vi "Read Unified Msg Set.vi"(11 "Base Setup in":refnum<class "Base Setup.lvclass">) -> (2 "Unified Msg Set":T1)   [LabVIEW 2025, in "jettl.lvlib" / "Setup.lvlib" / "Base Setup.lvclass"]
uses:
  Base Setup.lvclass
  Msg Set.ctl
  Msg/Msg.lvclass
  Base Setup.lvclass/Base Setup.ctl
  jettl.lvlib
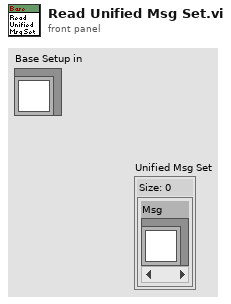
[diagram p1: front panel]
types:
  T1 = typedef "jettl.lvlib/Msg Set.ctl" = set{refnum<class "Msg.lvclass">}
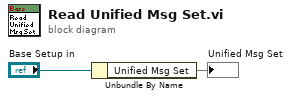
[diagram p0: block diagram]
diagram:
  n1 = Unbundle By Name("Base Setup in") -> ("Unified Msg Set"=→"Unified Msg Set":T1)
